vi "All TypeDefs.vi"() -> ()   [LabVIEW 2013, in "VRI.lvlib"]
uses:
  VRI.lvlib
  BITMAPINFO.ctl
  BITMAPINFOHEADER.ctl
  RGBQUAD.ctl
  PHCon ACQUIPARAMS.ctl
  PhCon SyncImaging.ctl
  Rect.ctl
  PHCon Time64.ctl
  PhInt CFA.ctl
  PHCon CAMERAOPTIONS.ctl
  PhCon VideoSystem.ctl
  PHCon IMRANGE.ctl
  PHCon CINESTATUS.ctl
  PhCon VerSel.ctl
  Point.ctl
  PhInt WBGAIN.ctl
  FilterCode.ctl
  PhInt IMPROCOPTIONS.ctl
  IMFILTER.ctl
  PnInt Setup.ctl
  PhFile PRANGE.ctl
  PhFile InfName.ctl
  PhFile HeadSaveOptions.ctl
  PhInt Algorithm.ctl
  PhInt Color.ctl
  PhCon GAD.ctl
  PhCon GDLO.ctl
  PhCon SDLO.ctl
  pEnable.ctl
  FileTypeIndex.ctl
  ACQUIPARAMS Display.ctl
  PhCon CAMERAID.ctl
  PhFile CmDesc.ctl
  PhFile ToneDesc.ctl
  PhFile SAVECINEINFO.ctl
  PhInt RECT.ctl
  PhInt TIME64.ctl
  TCU.ctl
  TC.ctl
panel:
  in  "TC":T1
  in  "TCU":T2
  in  "TIME64":T3
  in  "RECT":T4
  in  "SAVECINEINFO":T5
  in  "ToneDesc":T6
  in  "CmDesc":T7
  in  "CAMERAID":T8
  in  "ACQUIPARAMS Display":T9
  in  "FileTypeIndex":T10 items=["MIFILE_RAWCINE"=0, "MIFILE_CINE"=1, "MIFILE_AVI"=3, "MIFILE_TIFCINE"=4, "MIFILE_QTIME"=8, "SIFILE_TIF8"=-8, "SIFILE_TIF12"=-9, "SIFILE_TIF16"=-10, "SIFILE_RAW"=-25, "SIFILE_DNG"=-26, "SIFILE_DPX"=-27]
  in  "VideoSystem":T11 items=["VIDEOSYS_NTSC"=0, "VIDEOSYS_PAL"=1, "VIDEOSYS_720P60"=4, "VIDEOSYS_720P59DOT9"=12, "VIDEOSYS_720P50"=5, "VIDEOSYS_1080P30"=20, "VIDEOSYS_1080P29DOT9"=28, "VIDEOSYS_1080P25"=21, "VIDEOSYS_1080P24"=36, "VIDEOSYS_1080P23DOT9"=44, "VIDEOSYS_1080I30"=68, "VIDEOSYS_1080I29DOT9"=76, "VIDEOSYS_1080I25"=69, "VIDEOSYS_1080PSF30"=52, "VIDEOSYS_1080PSF29DOT9"=60, "VIDEOSYS_1080PSF25"=53, "VIDEOSYS_1080PSF24"=84, "VIDEOSYS_1080PSF23DOT9"=92]
  in  "SyncImaging":T12
  in  "pEnable":T13
  in  "SelectCode 2":T14=100 items=["SDLO_PHANTOM"=100, "SDLO_PHCON"=101, "SDLO_PHINT"=102, "SDLO_PHFILE"=103, "SDLO_PHSIG"=104, "SDLO_PHSIGV"=105, "SDLO_TORAM"=106]
  in  "SelectCode":T15=200 items=["GDLO_PHANTOM"=200, "GDLO_PHCON"=201, "GDLO_PHINT"=202, "GDLO_PHFILE"=203, "GDLO_PHSIG"=204, "GDLO_PHSIGV"=205, "GDLO_TORAM"=206]
  in  "Selection":u32(ring)=1 items=["GII_SOURCECAMERA"=1, "GII_SLICECOUNT"=2, "GII_SLICELIST"=3, "GII_VIRTUALCN"=4]
  in  "Sel":T16=1001 items=["GAD_TIMEXP"=1001, "GAD_TIME"=1002, "GAD_EXPOSURE"=1003, "GAD_RANGE1"=1004, "GAD_BINSIG"=1005, "GAD_ANASIG"=1006, "GAD_SMPTETC"=1007, "GAD_SMPTETCU"=1008]
  in  "Color":T17
  in  "CFA":T18 {"CFA" items=["CFA_NONE", "CFA_VRI", "CFA_VRIV6", "CFA_BAYER", "CFA_BAYERFLIP"]}
  in  "Algorithm":T19=5 items=["FAST_ALGORITHM"=1, "BEST_ALGORITHM"=5, "NO_DEMOSAICING"=6]
  in  "HeadSaveOptions":T20
  in  "InfName":T21 items=["GCI_CFA"=0, "GCI_FRAMERATE"=1, "GCI_EXPOSURE"=2, "GCI_AUTOEXPOSURE"=3, "GCI_REALBPP"=4, "GCI_CAMERASERIAL"=5, "GCI_HEADSERIAL0"=6, "GCI_HEADSERIAL1"=7, "GCI_HEADSERIAL2"=8, "GCI_HEADSERIAL3"=9, "GCI_TRIGTIMESEC"=10, "GCI_TRIGTIMEFR"=11, "GCI_ISFILECINE"=12, "GCI_IS16BPPCINE"=13, "GCI_ISCOLORCINE"=14, "GCI_ISMULTIHEADCINE"=15, "GCI_EXPOSURENS"=16, "GCI_EDREXPOSURENS"=17, "GCI_FRAMEDELAYNS"=19, "GCI_FROMFILETYPE"=20, "GCI_COMPRESSION"=21, "GCI_CAMERAVERSION"=22, "GCI_ROTATE"=23, "GCI_IMWIDTH"=24, "GCI_IMHEIGHT"=25, "GCI_IMWIDTHACQ"=26, "GCI_IMHEIGHTACQ"=27, "GCI_POSTTRIGGER"=28, "GCI_IMAGECOUNT"=29, "GCI_TOTALIMAGECOUNT"=30, "GCI_TRIGFRAME"=31, "GCI_AUTOEXPLEVEL"=32, "GCI_AUTOEXPTOP"=33, "GCI_AUTOEXPLEFT"=34, "GCI_AUTOEXPBOTTOM"=35, "GCI_AUTOEXPRIGHT"=36, "GCI_RECORDINGTIMEZONE"=37, "GCI_FIRSTIMAGENO"=38, "GCI_FIRSTMOVIEIMAGE"=39, "GCI_CINENAME"=40, "GCI_FRPSTEPS"=100, "GCI_FRP1X"=101, "GCI_FRP1Y"=102, "GCI_FRP2X"=103, "GCI_FRP2Y"=104, "GCI_FRP3X"=105, "GCI_FRP3Y"=106, "GCI_FRP4X"=107, "GCI_FRP4Y"=108, "GCI_WRITEERR"=109, "GCI_LENSDESCRIPTION"=110, "GCI_LENSAPERATURE"=111, "GCI_LENSFOCALLENGTH"=112, "GCI_WB"=200, "GCI_WBVIEW"=201, "GCI_BRIGHT"=202, "GCI_CONTRAST"=203, "GCI_GAMMA"=204, "GCI_GAMMAR"=223, "GCI_GAMMAB"=224, "GCI_SATURATION"=205, "GCI_HUE"=206, "GCI_FLIPH"=207, "GCI_FLIPV"=208, "GCI_FILTERCODE"=209, "GCI_IMFILTER"=210, "GCI_INTALGO"=211, "GCI_PEDESTALR"=212, "GCI_PEDESTALG"=213, "GCI_PEDESTALB"=214, "GCI_FLARE"=225, "GCI_CHROMA"=226, "GCI_TONE"=227, "GCI_ENABLEMATRICES"=228, "GCI_USERMATRIX"=229, "GCI_RESAMPLEACTIVE"=215, "GCI_RESAMPLEWIDTH"=216, "GCI_RESAMPLEHEIGHT"=217, "GCI_CROPACTIVE"=218, "GCI_CROPRECTANGLE"=219, "GCI_OFFSET16_8"=220, "GCI_GAIN16_8"=221, "GCI_DEMOSAICINGFUNCPTR"=222, "GCI_VFLIPVIEWACTIVE"=300, "GCI_MAXIMGSIZE"=400, "GCI_FRPIMGNOARRAY"=450, "GCI_FRPRATEARRAY"=451, "GCI_FRPSHAPEARRAY"=452, "GCI_TRIGTC"=470, "GCI_TRIGTCU"=471, "GCI_PBRATE"=472, "GCI_TCRATE"=473, "GCI_SAVERANGE"=500, "GCI_SAVEFILENAME"=501, "GCI_SAVEFILETYPE"=502, "GCI_SAVE16BIT"=503, "GCI_SAVEPACKED"=504, "GCI_SAVEXML"=505, "GCI_SAVESTAMPTIME"=506, "GCI_SAVEAVIFRAMERATE"=520, "GCI_SAVEAVICOMPRESSORLIST"=521, "GCI_SAVEAVICOMPRESSORINDEX"=522, "GCI_SAVEDPXLSB"=530, "GCI_SAVEDPXTO10BPS"=531, "GCI_SAVEDPXDATAPACKING"=532, "GCI_SAVEDPX10BITLOG"=533, "GCI_SAVEDPXEXPORTLOGLUT"=534, "GCI_SAVEDPX10BITLOGREFWHITE"=535, "GCI_SAVEDPX10BITLOGREFBLACK"=536, "GCI_SAVEDPX10BITLOGGAMMA"=537, "GCI_SAVEDPX10BITLOGFILMGAMMA"=538, "GCI_SAVEQTPLAYBACKRATE"=550, "GCI_SAVECCIQUALITY"=560, "GCI_UNCALIBRATEDIMAGE"=600, "GCI_NOPROCESSING"=601, "GCI_BADPIXELREPAIR"=602]
  in  "PRANGE":T22
  in  "IMFILTER":T23
  in  "Setup":T24
  in  "IMPROCOPTIONS":T27 {"FilterCode" items=["PREWITT_3X3_V"=1, "PREWITT_3X3_H"=2, "SOBEL_3X3_V"=3, "SOBEL_3X3_H"=4, "LAPLACIAN_3X3"=5, "LAPLACIAN_5X5"=6, "GAUSSIAN_3X3"=7, "GAUSSIAN_5X5"=8, "HIPASS_3x3"=9, "HIPASS_5x5"=10, "SHARPEN_3X3"=11, "USERFILTER"=-1]; "Rotate" min=-90 max=90 step=1; "Saturation" min=-100 max=100 step=1; "Contrast" min=-100 max=100 step=1; "Bright" min=-100 max=100 step=1}
  in  "FilterCode":T28 items=["PREWITT_3X3_V"=1, "PREWITT_3X3_H"=2, "SOBEL_3X3_V"=3, "SOBEL_3X3_H"=4, "LAPLACIAN_3X3"=5, "LAPLACIAN_5X5"=6, "GAUSSIAN_3X3"=7, "GAUSSIAN_5X5"=8, "HIPASS_3x3"=9, "HIPASS_5x5"=10, "SHARPEN_3X3"=11, "USERFILTER"=-1]
  in  "WBGAIN":T26
  in  "Point":T29
  in  "RGBQUAD":T30
  in  "VerSel":T31 items=["GV_CAMERA"=1, "GV_FIRMWARE"=2, "GV_FPGA"=3, "GV_PHCON"=4, "GV_CFA"=5, "GV_KERNEL"=6, "GV_MAGAZINE"=7]
  in  "Time64":T32 {"fractions" format="%32.0f"}
  in  "IMRANGE":T33
  in  "CINESTATUS":T34
  in  "CAMERAOPTIONS":T35 {"VideoSystem" items=["VIDEOSYS_NTSC"=0, "VIDEOSYS_PAL"=1, "VIDEOSYS_720P60"=4, "VIDEOSYS_720P59DOT9"=12, "VIDEOSYS_720P50"=5, "VIDEOSYS_1080P30"=20, "VIDEOSYS_1080P29DOT9"=28, "VIDEOSYS_1080P25"=21, "VIDEOSYS_1080P24"=36, "VIDEOSYS_1080P23DOT9"=44, "VIDEOSYS_1080I30"=68, "VIDEOSYS_1080I29DOT9"=76, "VIDEOSYS_1080I25"=69, "VIDEOSYS_1080PSF30"=52, "VIDEOSYS_1080PSF29DOT9"=60, "VIDEOSYS_1080PSF25"=53, "VIDEOSYS_1080PSF24"=84, "VIDEOSYS_1080PSF23DOT9"=92]}
  in  "ACQUIPARAMS":T36 {"CFA"."CFA" items=["CFA_NONE", "CFA_VRI", "CFA_VRIV6", "CFA_BAYER", "CFA_BAYERFLIP"]; "TriggerTime"."fractions" format="%32.0f"}
  in  "BITMAPINFOHEADER":T37
  out "pBMI":T38
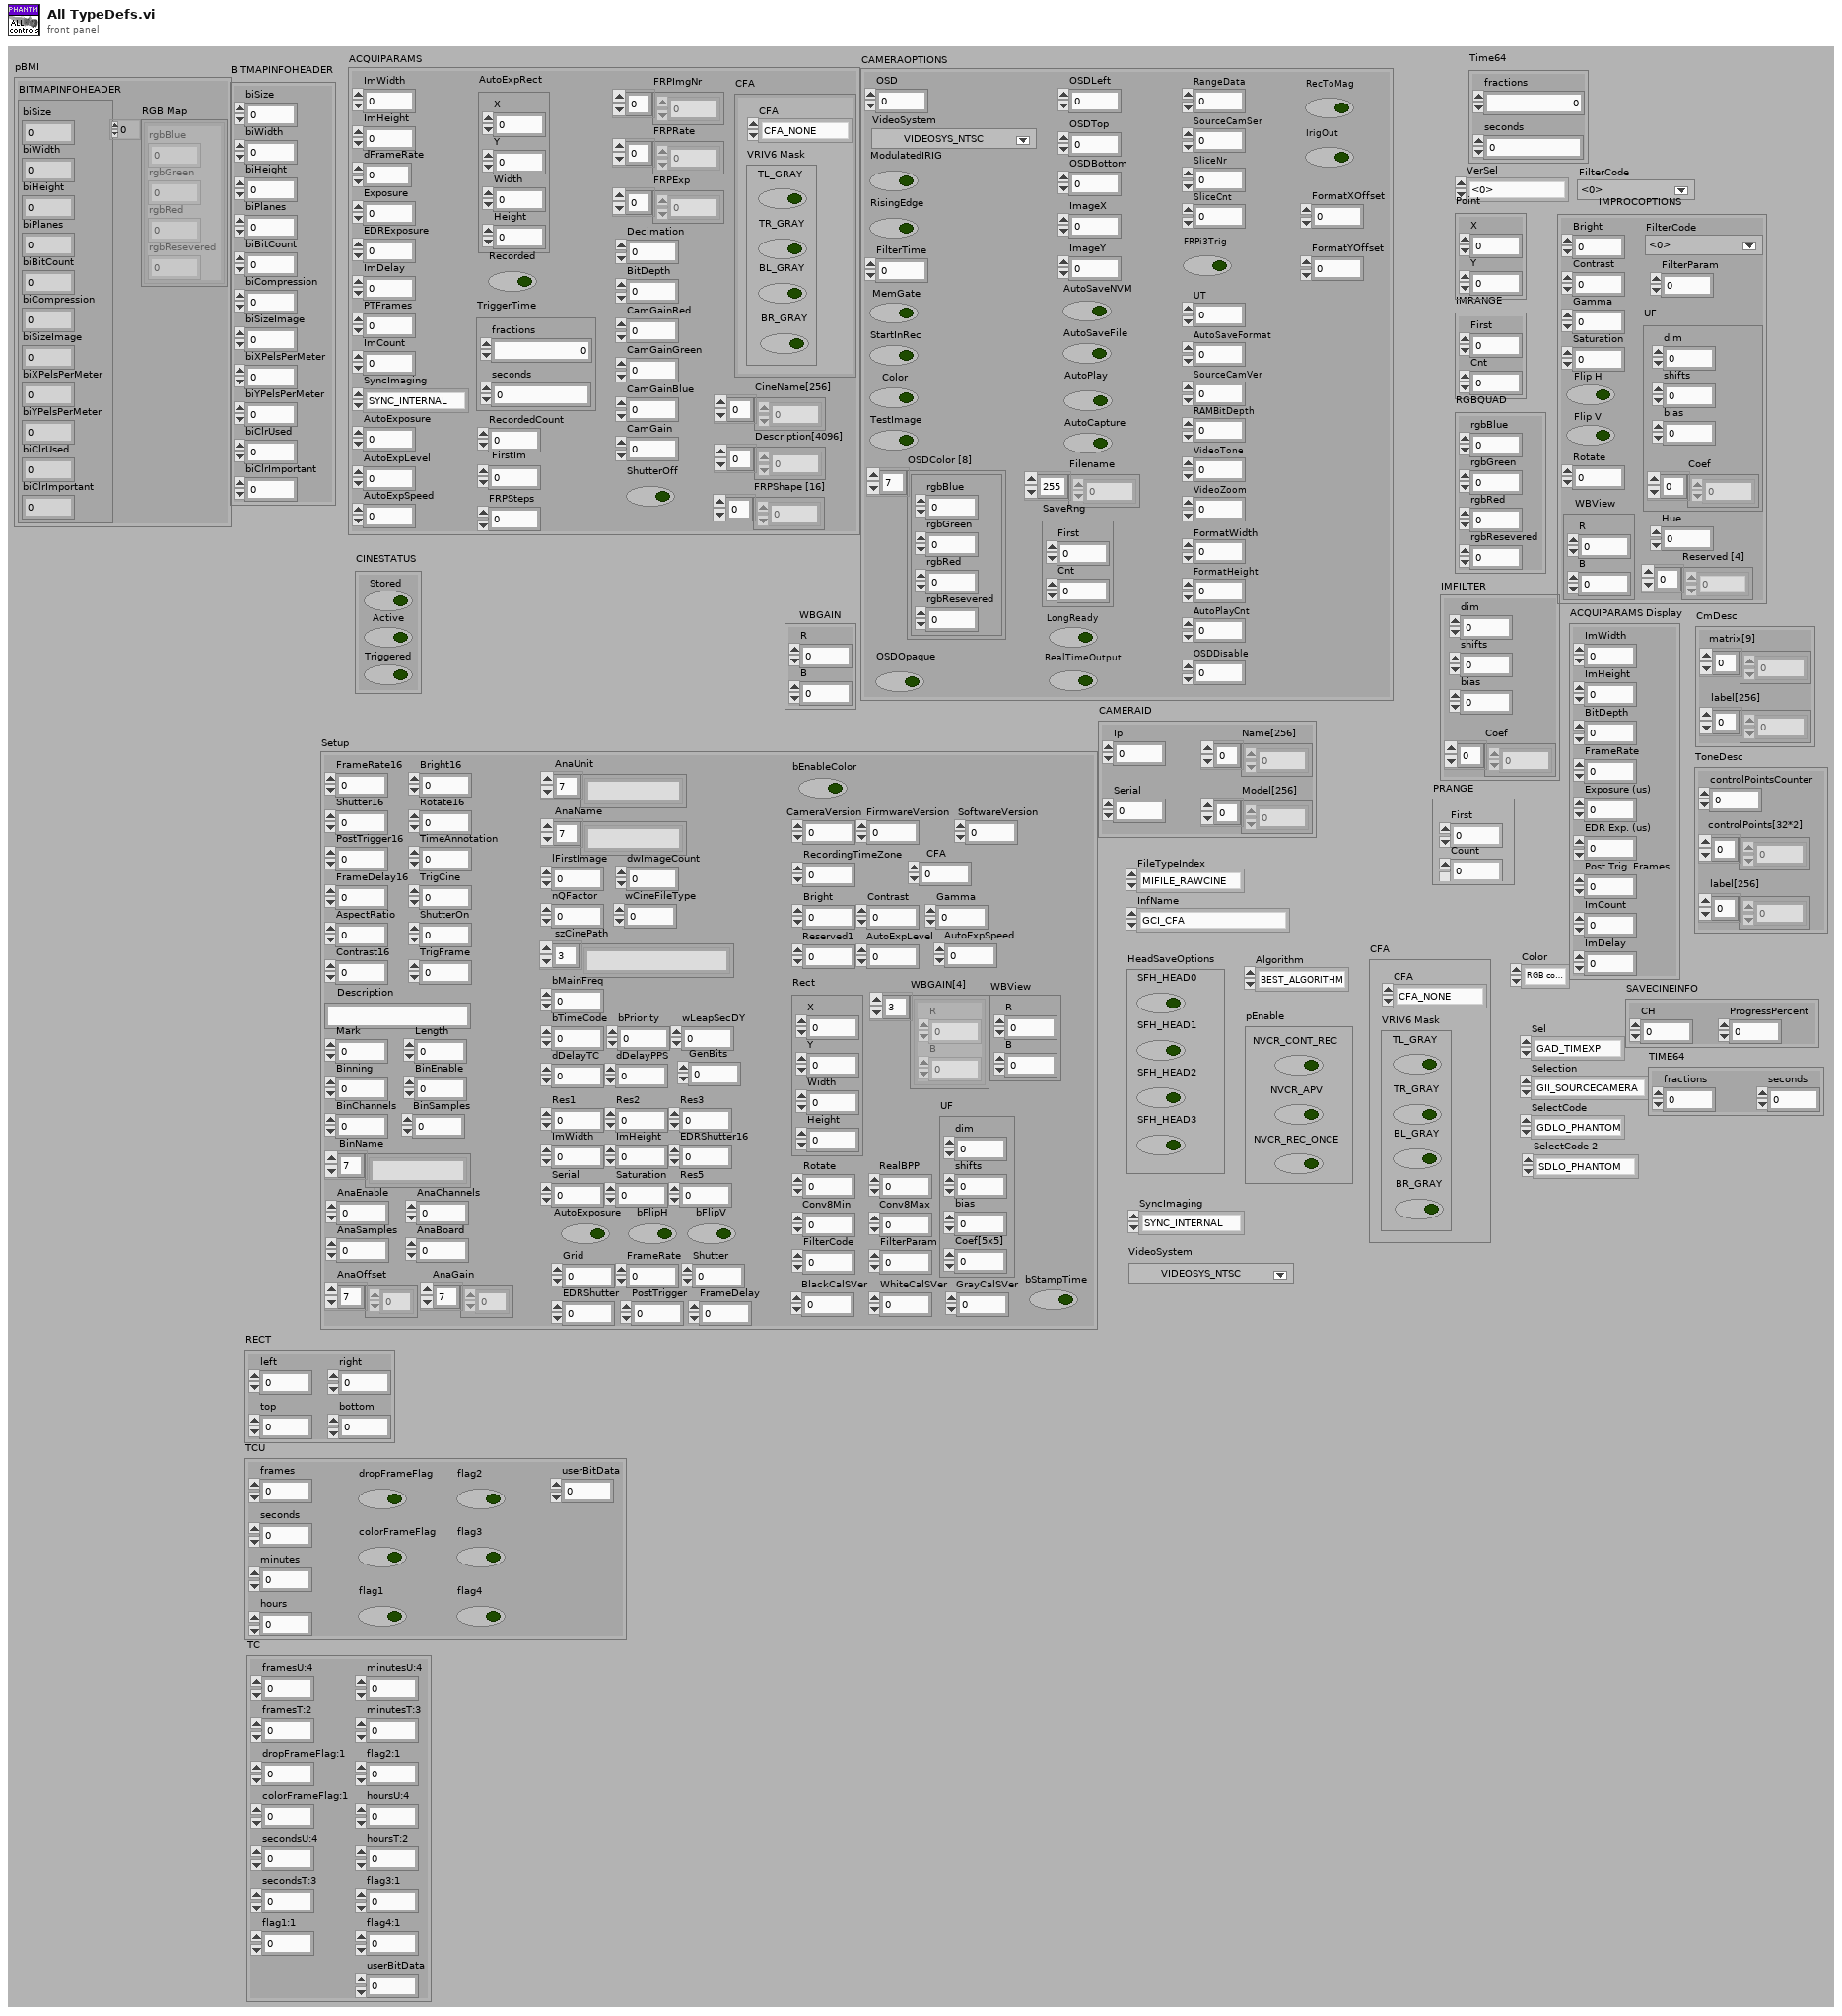
[diagram p1: front panel]
types:
  T1 = typedef "VRI.lvlib/TC.ctl" = cluster{"framesU:4":u8, "secondsT:3":u8, "framesT:2":u8, "dropFrameFlag:1":u8, "colorFrameFlag:1":u8, "secondsU:4":u8, "minutesU:4":u8, "flag1:1":u8, "minutesT:3":u8, "flag2:1":u8, "hoursU:4":u8, "hoursT:2":u8, "flag3:1":u8, "flag4:1":u8, "userBitData":u32}
  T2 = typedef "VRI.lvlib/TCU.ctl" = cluster{"frames":u32, "seconds":u32, "minutes":u32, "hours":u32, "userBitData":u32, "dropFrameFlag":bool, "colorFrameFlag":bool, "flag1":bool, "flag2":bool, "flag3":bool, "flag4":bool}
  T3 = typedef "VRI.lvlib/PhInt TIME64.ctl" = cluster{"fractions":u32, "seconds":u32}
  T4 = typedef "VRI.lvlib/PhInt RECT.ctl" = cluster{"left":i32, "top":i32, "right":i32, "bottom":i32}
  T5 = typedef "VRI.lvlib/PhFile SAVECINEINFO.ctl" = cluster{"CH":u32, "ProgressPercent":u32}
  T6 = typedef "VRI.lvlib/PhFile ToneDesc.ctl" = cluster{"controlPointsCounter":i32, "label[256]":u8[], "controlPoints[32*2]":dbl[]}
  T7 = typedef "VRI.lvlib/PhFile CmDesc.ctl" = cluster{"label[256]":u8[], "matrix[9]":dbl[]}
  T8 = typedef "VRI.lvlib/PhCon CAMERAID.ctl" = cluster{"Ip":u32, "Serial":u32, "Model[256]":u8[], "Name[256]":u8[]}
  T9 = typedef "VRI.lvlib/ACQUIPARAMS Display.ctl" = cluster{"ImWidth":u32, "ImHeight":u32, "FrameRate":u32, "Exposure (us)":u32, "EDR Exp. (us)":u32, "ImDelay":u32, "Post Trig. Frames":u32, "ImCount":u32, "BitDepth":u32}
  T10 = typedef "VRI.lvlib/FileTypeIndex.ctl" = i32
  T11 = typedef "VRI.lvlib/PhCon VideoSystem.ctl" = u32
  T12 = typedef "VRI.lvlib/PhCon SyncImaging.ctl" = enum32{"SYNC_INTERNAL", "SYNC_EXTERNAL", "SYNC_LOCKTOIRIG"}
  T13 = typedef "VRI.lvlib/pEnable.ctl" = cluster{"NVCR_CONT_REC":bool, "NVCR_APV":bool, "NVCR_REC_ONCE":bool}
  T14 = typedef "VRI.lvlib/PhCon SDLO.ctl" = u32
  T15 = typedef "VRI.lvlib/PhCon GDLO.ctl" = u16
  T16 = typedef "VRI.lvlib/PhCon GAD.ctl" = u32
  T17 = typedef "VRI.lvlib/PhInt Color.ctl" = enum32{"RGB converted to gray", "RED", "GREEN", "BLUE"}
  T18 = typedef "VRI.lvlib/PhInt CFA.ctl" = cluster{"CFA":u32, "VRIV6 Mask":cluster{"TL_GRAY":bool, "TR_GRAY":bool, "BL_GRAY":bool, "BR_GRAY":bool}}
  T19 = typedef "VRI.lvlib/PhInt Algorithm.ctl" = u32
  T20 = typedef "VRI.lvlib/PhFile HeadSaveOptions.ctl" = cluster{"SFH_HEAD0":bool, "SFH_HEAD1":bool, "SFH_HEAD2":bool, "SFH_HEAD3":bool}
  T21 = typedef "VRI.lvlib/PhFile InfName.ctl" = u32
  T22 = typedef "VRI.lvlib/PhFile PRANGE.ctl" = cluster{"First":u32, "Count":u32}
  T23 = typedef "VRI.lvlib/IMFILTER.ctl" = cluster{"dim":i32, "shifts":i32, "bias":i32, "Coef":i32[]}
  T24 = typedef "VRI.lvlib/PnInt Setup.ctl" = cluster{"FrameRate16":u32, "Shutter16":u32, "PostTrigger16":u32, "FrameDelay16":u32, "AspectRatio":u32, "Contrast16":u32, "Bright16":u32, "Rotate16":u8, "TimeAnnotation":u8, "TrigCine":u8, "TrigFrame":u8, "ShutterOn":u8, "Description":string, "Mark":u32, "Length":u32, "Binning":u32, "BinEnable":u32, "BinChannels":i16, "BinSamples":u32, "BinName":string[], "AnaEnable":u32, "AnaChannels":i16, "AnaSamples":u32, "AnaBoard":u32, "AnaOffset":i16[], "AnaGain":sgl[], "AnaUnit":string[], "AnaName":string[], "lFirstImage":i32, "dwImageCount":u32, "nQFactor":i16, "wCineFileType":u16, "szCinePath":string[], "bMainFreq":u16, "bTimeCode":u8, "bPriority":u8, "wLeapSecDY":dbl, "dDelayTC":dbl, "dDelayPPS":dbl, "GenBits":u16, "Res1":i32, "Res2":i32, "Res3":i32, "ImWidth":u16, "ImHeight":u16, "EDRShutter16":u16, "Serial":u32, "Saturation":i32, "Res5":i8, "AutoExposure":bool, "bFlipH":bool, "bFlipV":bool, "Grid":u32, "FrameRate":u32, "Shutter":u32, "EDRShutter":u32, "PostTrigger":u32, "FrameDelay":u32, "bEnableColor":bool, "CameraVersion":u32, "FirmwareVersion":u32, "SoftwareVersion":u32, "RecordingTimeZone":i32, "CFA":u32, "Bright":i32, "Contrast":i32, "Gamma":i32, "Reserved1":u32, "AutoExpLevel":u32, "AutoExpSpeed":u32, "Rect":T25, "WBGAIN[4]":T26[], "Rotate":i32, "WBView":T26, "RealBPP":u32, "Conv8Min":u32, "Conv8Max":u32, "FilterCode":i32, "FilterParam":i32, "UF":cluster{"dim":i32, "shifts":i32, "bias":i32, "Coef[5x5]":i32}, "BlackCalSVer":u32, "WhiteCalSVer":u32, "GrayCalSVer":u32, "bStampTime":bool}
  T25 = typedef "VRI.lvlib/Rect.ctl" = cluster{"X":i32, "Y":i32, "Width":i32, "Height":i32}
  T26 = typedef "VRI.lvlib/PhInt WBGAIN.ctl" = cluster{"R":sgl, "B":sgl}
  T27 = typedef "VRI.lvlib/PhInt IMPROCOPTIONS.ctl" = cluster{"Bright":i32, "Contrast":i32, "Gamma":sgl, "Saturation":i32, "Flip H":bool, "Flip V":bool, "Rotate":i32, "WBView":T26, "FilterCode":T28, "FilterParam":i32, "UF":T23, "Hue":i32, "Reserved [4]":i32[]}
  T28 = typedef "VRI.lvlib/FilterCode.ctl" = i32
  T29 = typedef "VRI.lvlib/Point.ctl" = cluster{"X":i32, "Y":i32}
  T30 = typedef "VRI.lvlib/RGBQUAD.ctl" = cluster{"rgbBlue":u8, "rgbGreen":u8, "rgbRed":u8, "rgbResevered":u8}
  T31 = typedef "VRI.lvlib/PhCon VerSel.ctl" = u16
  T32 = typedef "VRI.lvlib/PHCon Time64.ctl" = cluster{"fractions":u32, "seconds":u32}
  T33 = typedef "VRI.lvlib/PHCon IMRANGE.ctl" = cluster{"First":i32, "Cnt":u32}
  T34 = typedef "VRI.lvlib/PHCon CINESTATUS.ctl" = cluster{"Stored":bool, "Active":bool, "Triggered":bool}
  T35 = typedef "VRI.lvlib/PHCon CAMERAOPTIONS.ctl" = cluster{"OSD":u32, "VideoSystem":T11, "ModulatedIRIG":bool, "RisingEdge":bool, "FilterTime":u32, "MemGate":bool, "StartInRec":bool, "Color":bool, "TestImage":bool, "OSDColor [8]":T30[], "OSDOpaque":bool, "OSDLeft":i32, "OSDTop":i32, "OSDBottom":i32, "ImageX":i32, "ImageY":i32, "AutoSaveNVM":bool, "AutoSaveFile":bool, "AutoPlay":bool, "AutoCapture":bool, "Filename":u8[], "SaveRng":T33, "LongReady":bool, "RealTimeOutput":bool, "RangeData":u32, "SourceCamSer":u32, "SliceNr":u32, "SliceCnt":u32, "FRPi3Trig":bool, "UT":u32, "AutoSaveFormat":i8, "SourceCamVer":u32, "RAMBitDepth":u32, "VideoTone":i32, "VideoZoom":i32, "FormatWidth":i32, "FormatHeight":i32, "AutoPlayCnt":u32, "OSDDisable":u32, "RecToMag":bool, "IrigOut":bool, "FormatXOffset":i32, "FormatYOffset":i32}
  T36 = typedef "VRI.lvlib/PHCon ACQUIPARAMS.ctl" = cluster{"ImWidth":u32, "ImHeight":u32, "(deprecated)FrameRateInt":u32, "Exposure":u32, "EDRExposure":u32, "ImDelay":u32, "PTFrames":u32, "ImCount":u32, "SyncImaging":T12, "AutoExposure":u32, "AutoExpLevel":u32, "AutoExpSpeed":u32, "AutoExpRect":T25, "Recorded":bool, "TriggerTime":T32, "RecordedCount":u32, "FirstIm":i32, "FRPSteps":u32, "FRPImgNr":i32[], "FRPRate":u32[], "FRPExp":u32[], "Decimation":u32, "BitDepth":u32, "CamGainRed":u32, "CamGainGreen":u32, "CamGainBlue":u32, "CamGain":u32, "ShutterOff":bool, "CFA":T18, "CineName[256]":u8[], "Description[4096]":u8[], "FRPShape [16]":u32[], "dFrameRate":dbl}
  T37 = typedef "VRI.lvlib/BITMAPINFOHEADER.ctl" = cluster{"biSize":u32, "biWidth":i32, "biHeight":i32, "biPlanes":u16, "biBitCount":u16, "biCompression":u32, "biSizeImage":u32, "biXPelsPerMeter":i32, "biYPelsPerMeter":i32, "biClrUsed":u32, "biClrImportant":u32}
  T38 = typedef "VRI.lvlib/BITMAPINFO.ctl" = cluster{"BITMAPINFOHEADER":T37, "RGB Map":T30[]}
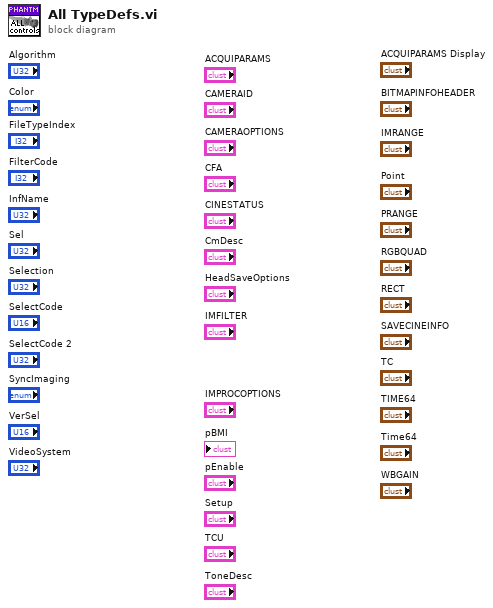
[diagram p0: block diagram]
diagram:
